vi "Get Default Name.vi"(8 "error in (no error)":errorcluster, 11 "Interlock Sample in":refnum<class "Interlock Sample.lvclass">) -> (0 "error out":errorcluster, 2 "Name":string, 3 "Interlock Sample out":refnum<class "Interlock Sample.lvclass">)   [LabVIEW 2015, in "cRIO-Carbondioxide.lvlib" / "Interlock Sample.lvclass"]
uses:
  Interlock Sample.lvclass
  Interlock Sample.lvclass/Interlock Sample.ctl
  <resource>/objmgr/ni.var.rc
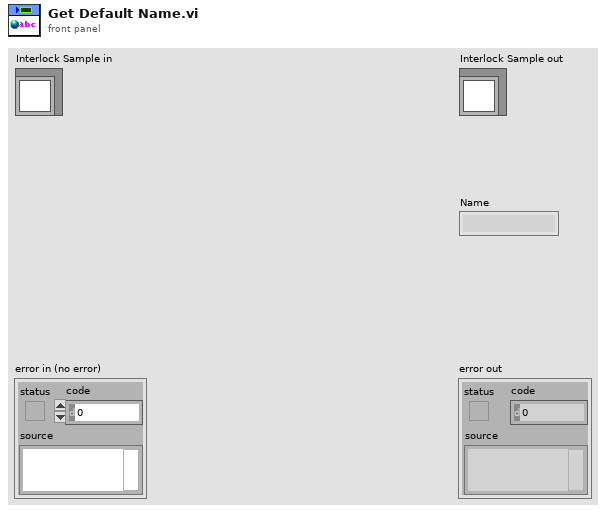
[diagram p1: front panel]
types:
  T1 = typedef "Sample Container.ctl" = cluster{"Sample In":refnum<k21>, "Sample Name":refnum<k21>, "Ti Cathode":refnum<k21>, "SampleQ":refnum<queue>}
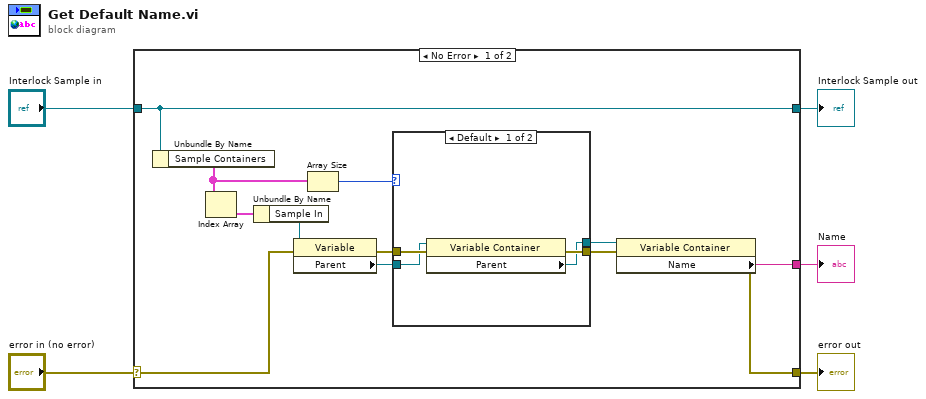
[diagram p0: block diagram]
diagram:
  n1 = case shown="No Error" "error in (no error)" {
    selector: "error in (no error)" -> [w15 w25]
    tunnel: [w16 w25] -> w4
    tunnel: [w17 w24] -> w2
    tunnel: "Interlock Sample in" -> [w17 w24]
    tunnel: [w14 _] -> w1
    frame No Error {
      n2 = Unbundle By Name(w17) -> ("Sample Containers"=w11:T1[])
      n3 = Index Array(array=w11) -> (element=w13:T1)  [unwired: 1 in]
      n4 = Unbundle By Name(w13) -> ("Sample In"=w12:refnum<k21>)
      n5 = property class="Variable"(reference=w12, error in=w15) -> (error out=w9:errorcluster, "Parent"=w6:refnum<k21>)  [unwired: 1 out]
      n6 = Array Size(array=w11) -> (size(s)=w10:i32)
      n7 = case shown="Default" w10 {
        tunnel: w9 -> [w21 w23]
        tunnel: [w19 w23] -> w8
        tunnel: [w18 w22] -> w7
        tunnel: w6 -> [w20 w22]
        frame Default {
          n8 = property class="Variable Container"(reference=w20, error in=w21) -> (error out=w19:errorcluster, "Parent"=w18:refnum<k21>)  [unwired: 1 out]
        }
        frame 1 {
        }
      }
      n9 = property class="Variable Container"(reference=w7, error in=w8) -> (error out=w16:errorcluster, "Name"=w14:string)  [unwired: 1 out]
    }
    frame Error {
    }
  }
  "error out" <- w4
  "Interlock Sample out" <- w2
  "Name" <- w1
